vi "To Pretty String (Null).vi"(5 "indent":i32, 11 "error in (no error)":errorcluster) -> (4 "String":string, 15 "error out":errorcluster)   [LabVIEW 2017, in "Variant JSON API.lvlib"]
doc: "Flattens the given JSON data to a string."
uses:
  Variant JSON API.lvlib
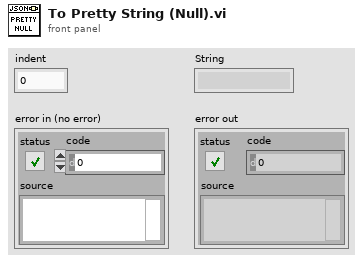
[diagram p1: front panel]
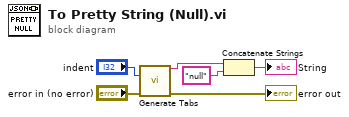
[diagram p0: block diagram]
diagram:
  n1 = call "Generate Tabs.vi"("indent"="indent", "error in (no error)"="error in (no error)") -> ("Tabs"=w5:string, "error out"=→"error out":errorcluster)  [unwired: 12 in]
  n2 = Concatenate Strings(w5, "null" ("String")) -> (→"String":string)
